vi "Simple XBox Tester.vi"() -> ()   [LabVIEW 2020]
uses:
  Joystick/XBox POV.ctl
  Joystick/XBox Axis.ctl
  Joystick/XBox Button.ctl
  Joystick/Joystick/Joystick.lvclass/Joystick.ctl
  96fb2d79-bee8-4724-a526-d2db6b4a61d2.vi
  47c4be0d-5e25-48ec-a32c-c70f933655d3.vi
  783c63d9-0c19-4758-a0b5-0cf0f4335bd0.vi
  Joystick/Joystick/_POV Value.vi
  Joystick/Joystick/_Axis Value.vi
  Joystick/Joystick/_Button Value.vi
  Joystick/Joystick/Joystick.lvclass
  Joystick/Joystick.lvlib
panel:
  out "RS Button":bool
  out "LS Button":bool
  out "RTrigger":dbl(slide) scale=0.0..32768.0
  out "LTrigger":dbl(slide) scale=0.0..32768.0
  out "RBumper":bool
  out "LBumper":bool
  out "Start":bool
  out "Back":bool
  out "A":bool
  out "B":bool
  out "Y":bool
  out "X":bool
  out "D-Pad":cluster{"X":dbl, "Y":dbl}[](graph)
  out "Right Stick":cluster{"X":dbl, "Y":dbl}[](graph)
  out "Left Stick":cluster{"X":dbl, "Y":dbl}[](graph)
  in  "Joystick Index":i32
  # "*** Change Index to use a different available joystick/gamepad ***"
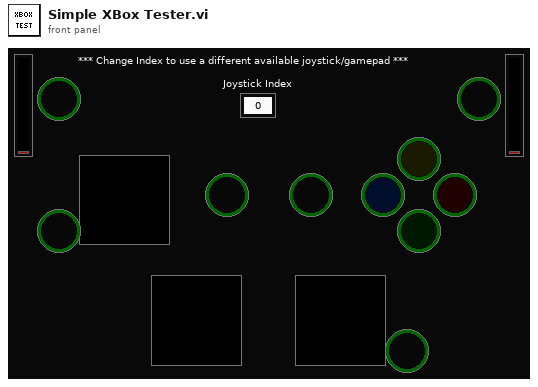
[diagram p1: front panel]
types:
  T1 = typedef "Joystick.lvlib/XBox POV.ctl" = enum16{"DPad"}
  T2 = typedef "Joystick.lvlib/XBox Button.ctl" = enum16{"A", "B", "X", "Y", "LB", "RB", "Back", "Start", "LS", "RS"}
  T3 = typedef "Joystick.lvlib/XBox Axis.ctl" = enum16{"Left Stick X", "Left Stick Y", "Triggers", "Right Stick X", "Right Stick Y"}
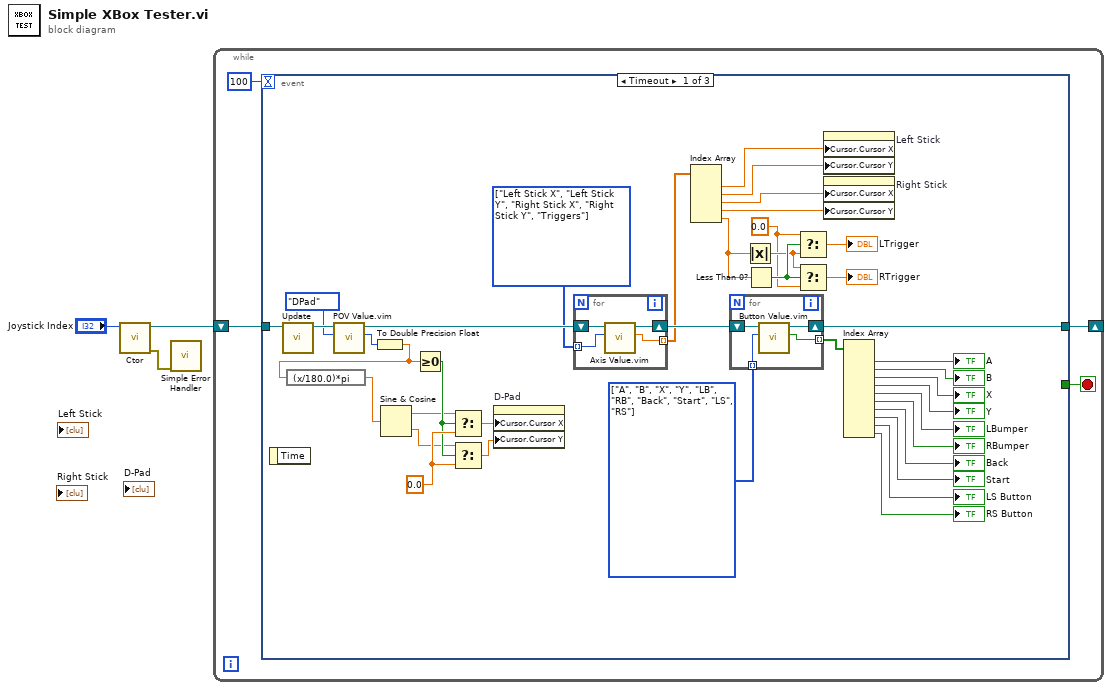
[diagram p0: block diagram]
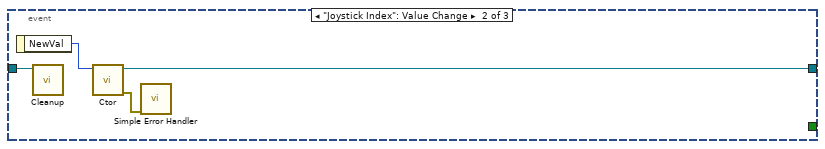
[diagram p2: hidden frame]
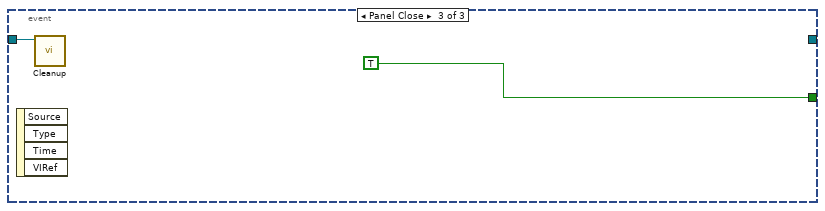
[diagram p3: hidden frame]
diagram:
  n1 = call "Ctor.vi"("Joystick Index"="Joystick Index") -> ("error out"=w1:errorcluster, "Joystick out"=w2:refnum<class "Joystick.lvclass">)  [unwired: 9 in]
  n2 = call <vilib>:"Simple Error Handler.vi"("error in (no error)"=w1) -> ()  [unwired: 4 in, 5 out]
  n3 = while {
    shift-right: [w4] -> _
    shift-left: w2 -> [w6]
    stop <- w5 stop-if-true
    n4 = event shown="[0] Timeout" {
      selector: _ -> [_ _ _]
      dyn-events: _ -> [_ _ _]
      timeout: 100 -> [_ _ _]
      tunnel: w6 -> [w46 w58 w59]
      tunnel: [_ _ TRUE] -> w5
      tunnel: [w28 w56 _] -> w4
      event Timeout {
        w13 = 0.0
        w19 = 0.0
        w40 = T2[] [enum."A", enum."B", enum."X", enum."Y", enum."LB", enum."RB", enum."Back", enum."Start", enum."LS", enum."RS"] items=["A", "B", "X", "Y", "LB", "RB", "Back", "Start", "LS", "RS"]
        w42 = T3[] [enum."Left Stick X", enum."Left Stick Y", enum."Right Stick X", enum."Right Stick Y", enum."Triggers"] items=["Left Stick X", "Left Stick Y", "Triggers", "Right Stick X", "Right Stick Y"]
        n5 = event-data() -> ()  [unwired: 1 in, 1 out]
        n6 = call "Update.vi"("Joystick in"=w46) -> ("Joystick out"=w45:refnum<class "Joystick.lvclass">)  [unwired: 9 in, 1 out]
        n7 = call "POV Value.vim"("POV or Index"=XBox_POV."DPad" ("XBox POV"), "Joystick in"=w45) -> ("Value"=w16:i32, "Joystick out"=w43:refnum<class "Joystick.lvclass">)  [unwired: 7 in, 1 out]
        n8 = To Double Precision Float(number=w16) -> (double precision float=w14:dbl)
        n9 = expression code="(x/180.0)*pi" ("degrees to radians")(w14) -> (w15:dbl)
        n10 = Sine & Cosine(0:w15) -> (1:w11:dbl, 2:w10:dbl)
        n11 = Greater Or Equal To 0?(x=w14) -> (x >= 0?=w12:bool)
        n12 = Select(t=w11, s=w12, f=w13) -> (s? t:f=w9:dbl)
        n13 = Select(t=w10, s=w12, f=w13) -> (s? t:f=w8:dbl)
        n14 = property on="D-Pad" class="XYGraph (strict)"("Cursor.Cursor X"=w9, "Cursor.Cursor Y"=w8) -> ()  [unwired: 2 in, 2 out]
        n15 = for {
          shift-right: [w52] -> w41
          shift-left: w43 -> [w54]
          tunnel: w42 -> [w53] mode=indexing
          tunnel: [w51] -> w27 mode=indexing
          n16 = call "Axis Value.vim"("Axis or Index"=w53, "Joystick in"=w54) -> ("Axis Value"=w51:dbl, "Joystick out"=w52:refnum<class "Joystick.lvclass">)  [unwired: 7 in, 1 out]
        }
        n17 = Index Array(array=w27) -> (element #1=w26:dbl, element #2=w25:dbl, element #3=w24:dbl, element #4=w23:dbl, element #5=w22:dbl)  [unwired: 5 in]
        n18 = for {
          shift-right: [w48] -> w28
          shift-left: w41 -> [w50]
          tunnel: w40 -> [w49] mode=indexing
          tunnel: [w47] -> w39 mode=indexing
          n19 = call "Button Value.vim"("Button or Index"=w49, "Joystick in"=w50) -> ("Value"=w47:bool, "Joystick out"=w48:refnum<class "Joystick.lvclass">)  [unwired: 7 in, 1 out]
        }
        n20 = Absolute Value(x=w22) -> (abs(x)=w20:dbl)
        n21 = Less Than 0?(x=w22) -> (x < 0?=w21:bool)
        n22 = Select(t=w19, s=w21, f=w20) -> (s? t:f=→"LTrigger":dbl)
        n23 = Select(t=w20, s=w21, f=w19) -> (s? t:f=→"RTrigger":dbl)
        n24 = property on="Left Stick" class="XYGraph (strict)"("Cursor.Cursor X"=w26, "Cursor.Cursor Y"=w25) -> ()  [unwired: 2 in, 2 out]
        n25 = property on="Right Stick" class="XYGraph (strict)"("Cursor.Cursor X"=w24, "Cursor.Cursor Y"=w23) -> ()  [unwired: 2 in, 2 out]
        n26 = Index Array(array=w39) -> (element #1=→"A":bool, element #2=→"B":bool, element #3=→"X":bool, element #4=→"Y":bool, element #5=→"LBumper":bool, element #6=→"RBumper":bool, element #7=→"Back":bool, element #8=→"Start":bool, element #9=→"LS Button":bool, element #10=→"RS Button":bool)  [unwired: 10 in]
      }
      event "Joystick Index": Value Change {
        n27 = event-data() -> ("NewVal"=w57:i32)  [unwired: 1 in]
        n28 = call "Cleanup.vi"("Joystick in"=w58) -> ()  [unwired: 10 in, 1 out]
        n29 = call "Ctor.vi"("Joystick Index"=w57) -> ("error out"=w55:errorcluster, "Joystick out"=w56:refnum<class "Joystick.lvclass">)  [unwired: 9 in]
        n30 = call <vilib>:"Simple Error Handler.vi"("error in (no error)"=w55) -> ()  [unwired: 4 in, 5 out]
      }
      event Panel Close {
        n31 = event-data() -> ()  [unwired: 1 in, 4 out]
        n32 = call "Cleanup.vi"("Joystick in"=w59) -> ()  [unwired: 10 in, 1 out]
      }
    }
  }
